vi "CVT String IndexWrite.vi"(3 "error in (no error)":errorcluster, 4 "Value":string, 5 "Tag Index":i32) -> (0 "error out":errorcluster)   [LabVIEW 2014, in "QwaveSys Raspberry Pi Library.lvlib"]
uses:
  _SubVIs/TypeDefs/cvt_MemBlock Methods.ctl
  QwaveSys Raspberry Pi Library.lvlib
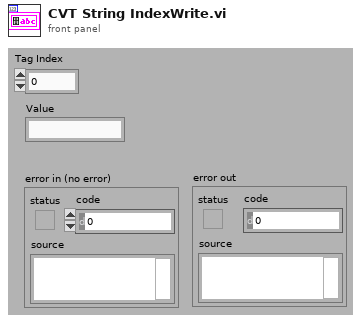
[diagram p1: front panel]
types:
  T1 = typedef "QwaveSys Raspberry Pi Library.lvlib/cvt_MemBlock Methods.ctl" = enum16{"init", "read", "readall", "write"}
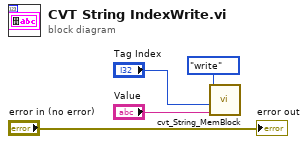
[diagram p0: block diagram]
diagram:
  n1 = call "cvt_String_MemBlock.vi"("Value"="Value", "Index"="Tag Index", "Method"=cvt_MemBlock_Methods."write") -> ()  [unwired: 1 in, 8 out]
  "error out" <- "error in (no error)"
